vi "FPGA_1R_ADC_1W_DAC_2AI_Phaseunwrap_Oct.vi"() -> ()   [LabVIEW 2019]
uses:
  <vilib>/rvi/FXPMathLib/FxpSinAndCos/subVIs/nifxpmath_SinAndCos_SimConfig.ctl
  <vilib>/rvi/FXPMathLib/FxpAtan2/subVIs/nifxpmath_Atan2_SimConfig.ctl
  <vilib>/rvi/Emulation/niFpgaGetClockAttributes.vi
  <vilib>/rvi/Emulation/niFpgaSctlEmulationGetInTimedLoop.vi
  <vilib>/rvi/Emulation/niFpgaEmulationReportErrorSimple.vi
  <vilib>/rvi/eio/common/nirviEmuTemplateMethod_errors.vi
  <vilib>/rvi/Emulation/niFpgaCriticalErrorInLSC.vi
  <vilib>/rvi/FXPMathLib/FxpSinAndCos/simVIs/DllFxpSinAndCosTemp_sub.vi
  <vilib>/rvi/FXPMathLib/FxpAtan2/simVIs/DllFxpAtan2Temp_sub.vi
  <vilib>/eio/EIONode/EIONode.xnode
  <vilib>/rvi/FXPMathLib/basic elements/FxpAddSub/XNode/nifxpmath_AddSub.xnode
  <vilib>/rvi/FXPMathLib/FxpSinAndCos/XNode/nifxpmath_SinAndCos.xnode
  <vilib>/rvi/FXPMathLib/FxpMul/XNode/nifxpmath_Multiplier.xnode
  <vilib>/rvi/FXPMathLib/FxpSub/XNode/nifxpmath_Sub.xnode
  <vilib>/rvi/FXPMathLib/FxpAdd/XNode/nifxpmath_Add.xnode
  <vilib>/rvi/FXPMathLib/FxpAtan2/XNode/nifxpmath_Atan2.xnode
  <vilib>/rvi/FXPMathLib/basic elements/FxpDiscreteDelay/XNode/nifxpmath_DiscreteDelay.xnode
  <vilib>/rvi/FXPMathLib/sim/FxpSim.dll
panel:
  out "unwrapped phase":fxp<+/-,47,33>
  out "X":fxp<+/-,64,28>
  out "Y":fxp<+/-,64,28>
  in  "1/a":fxp<+/-,16,2>
  in  "1/b":fxp<+/-,16,2>
  in  "x0":fxp<+/-,16,2>
  in  "y0":fxp<+/-,16,2>
  in  "theta":fxp<+/-,16,2>
  out "IFO Loop ticks actual":u32
  in  "IFO Timer Ticks":u32 caption="IFO Loop ticks desired"
  out "n":i32
  out "PD2":u16
  in  "?":bool
  out "PD1":u16
  in  "DAQ stop":bool
  out "ADC Read":bool[](array[boolean])
  out "DAQ TICKS":u32
  in  "DAQ WAIT TICKS":u32=800
  in  "DAC 1 write":bool[](array[boolean])=[FALSE, FALSE, FALSE, FALSE, FALSE, FALSE, FALSE, FALSE, FALSE, FALSE, FALSE, FALSE, FALSE, FALSE, FALSE, FALSE]
  out "XFWD":bool
  out "XREV":bool
  out "YFWD":bool
  out "YREV":bool
  in  "Limit flag stop":bool
  in  "ENC stop":bool
  out "Encoder A Ref":bool
  out "Encoder B Ref":bool
  out "Encoder A":i32
  out "Encoder B":i32
  in  "2^n avg_window":i16=8
  out "ENCODER OVERFLOW":bool
  out "ENCODER TICKS":u32
  in  "ENCODER TICK SETPOINT":u32=8
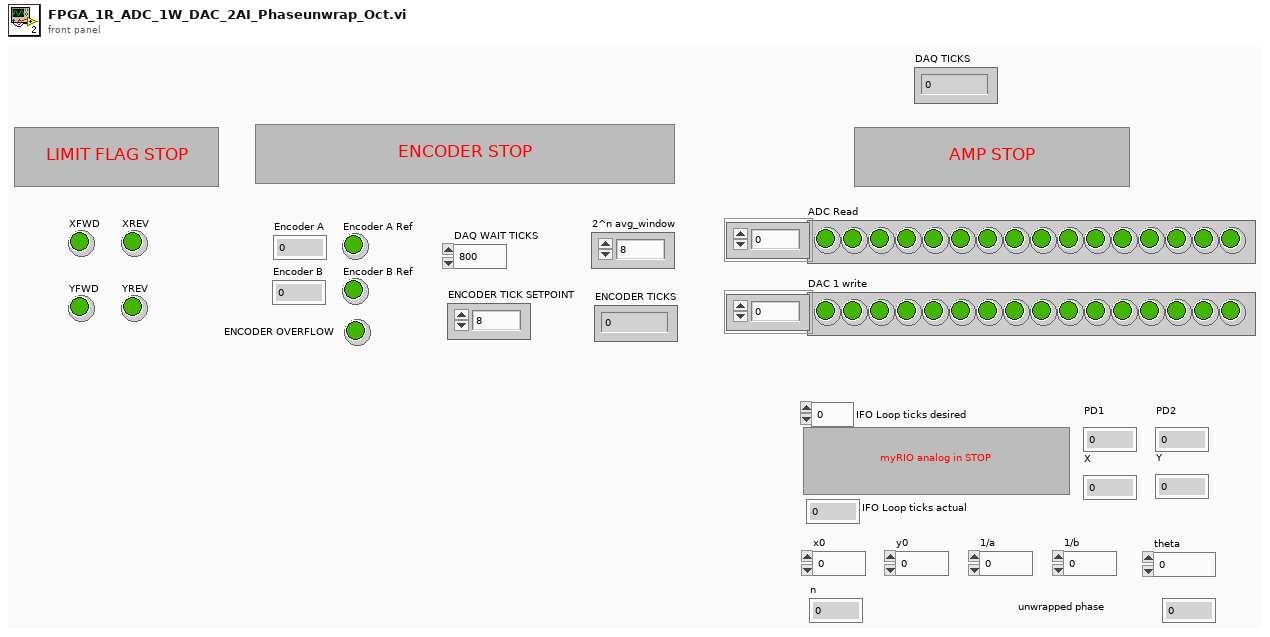
[diagram p1: front panel]
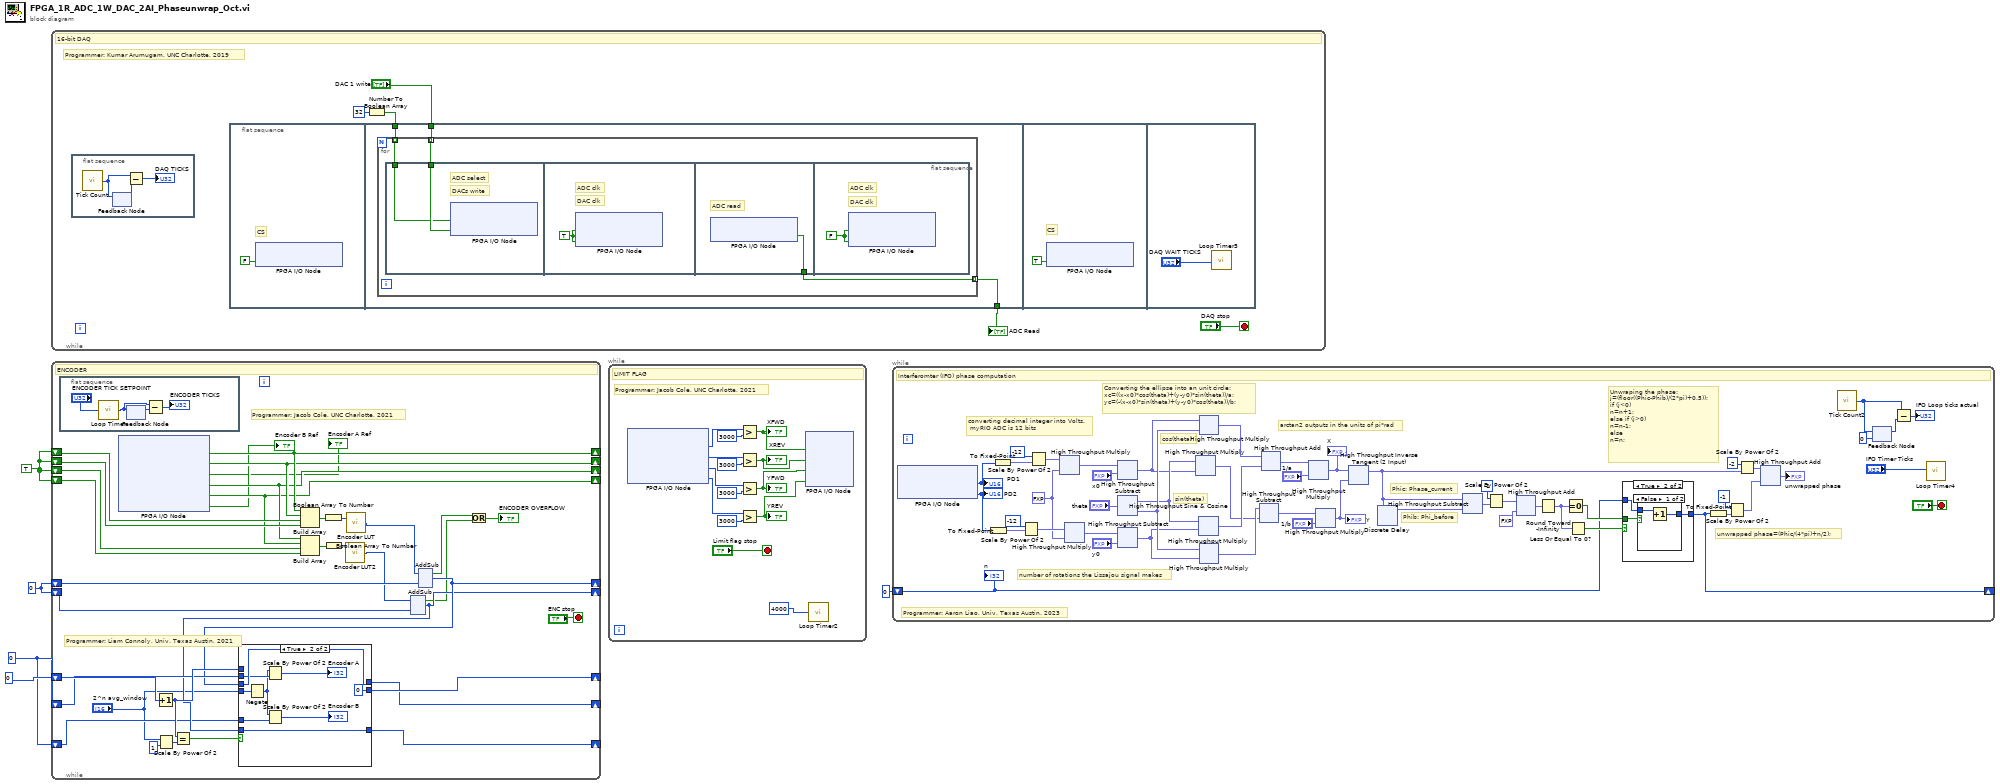
[diagram p0: block diagram]
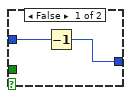
[diagram p2: hidden frame]
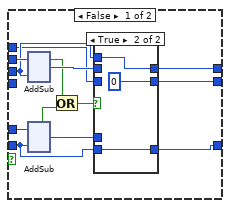
[diagram p4: hidden frame]
diagram:
  w2 = i64 0
  w4 = TRUE
  w5 = 0
  n1 = while {
    stop <- "DAQ stop" stop-if-true
    # "Programmer: Kumar Arumugam, UNC Charlotte, 2019"
    # "16-bit DAQ"
    n2 = flat-sequence {
      frame #0 {
        n3 = call "Tick Count"() -> ("Tick Count(Ticks)"=w27:u32)
        n4 = feedback #1() -> (w26:u32)  [unwired: 1 in]
        n5 = feedback-in #1(w27) -> ()
        n6 = Subtract(x=w27, y=w26) -> (x-y=→"DAQ TICKS":u32)
      }
    }
    n7 = flat-sequence {
      tunnel: "DAC 1 write" -> [w14]
      tunnel: w8 -> [w13]
      tunnel: [w12] -> w6
      frame #0 {
        # "CS"
        n8 = xnode "FPGA I/O Node"("ConnectorA/DIO4"=FALSE) -> ()  [unwired: 1 in, 1 out]
      }
      frame #1 {
        n9 = for {
          tunnel: w14 -> [w17] mode=indexing
          tunnel: [w16] -> w12 mode=indexing
          tunnel: w13 -> [w15] mode=indexing
          n10 = flat-sequence {
            tunnel: w17 -> [w19]
            tunnel: w15 -> [w18]
            tunnel: [w21] -> w16
            frame #0 {
              # "DACs write"
              # "ADC select"
              n11 = xnode "FPGA I/O Node"("ConnectorA/DIO2"=w18, "ConnectorA/DIO6"=w19) -> ()  [unwired: 2 in, 2 out]
            }
            frame #1 {
              w20 = TRUE ("ConnectorA/DIO3")
              # "DAC clk"
              # "ADC clk"
              n12 = xnode "FPGA I/O Node"("ConnectorA/DIO3"=w20, "ConnectorA/DIO5"=w20) -> ()  [unwired: 2 in, 2 out]
            }
            frame #2 {
              # "ADC read"
              n13 = xnode "FPGA I/O Node"() -> ("ConnectorA/DIO1"=w21:bool)  [unwired: 1 in, 1 out]
            }
            frame #3 {
              w22 = FALSE ("ConnectorA/DIO3")
              # "DAC clk"
              # "ADC clk"
              n14 = xnode "FPGA I/O Node"("ConnectorA/DIO3"=w22, "ConnectorA/DIO5"=w22) -> ()  [unwired: 2 in, 2 out]
            }
          }
        }
      }
      frame #2 {
        # "CS"
        n15 = xnode "FPGA I/O Node"("ConnectorA/DIO4"=TRUE) -> ()  [unwired: 1 in, 1 out]
      }
      frame #3 {
        n16 = call "Loop Timer3"("Count(Ticks)"="DAQ WAIT TICKS") -> ()  [unwired: 1 out]
      }
    }
    n17 = Number To Boolean Array(number=u16 32) -> (Boolean array=w8:bool[])
    "ADC Read" <- w6
  }
  n18 = while {
    shift-right: [w41] -> _
    shift-left: w5 -> [w39]
    shift-right: [w55] -> _
    shift-left: w4 -> [w61]
    shift-right: [w54] -> _
    shift-left: w4 -> [w58]
    shift-right: [w53] -> _
    shift-left: w4 -> [w57]
    shift-right: [w52] -> _
    shift-left: w4 -> [w56]
    shift-right: [w36] -> _
    shift-left: w5 -> [w37]
    shift-right: [w44] -> _
    shift-left: i16 0 -> [w47]
    shift-right: [w43] -> _
    shift-left: w2 -> [w42]
    shift-right: [w35] -> _
    shift-left: w2 -> [w34]
    stop <- "ENC stop" stop-if-true
    # "Programmer: Liam Connoly, Univ. Texas Austin, 2021"
    # "Programmer: Jacob Cole, UNC Charlotte, 2021"
    # "ENCODER"
    n19 = flat-sequence {
      frame #0 {
        n20 = call "Loop Timer"("Count(Ticks)"="ENCODER TICK SETPOINT") -> ("Tick Count(Ticks)"=w65:u32)
        n21 = feedback #2() -> (w64:u32)  [unwired: 1 in]
        n22 = feedback-in #2(w65) -> ()
        n23 = Subtract(x=w65, y=w64) -> (x-y=→"ENCODER TICKS":u32)
      }
    }
    n24 = xnode "FPGA I/O Node"() -> ("ConnectorA/DIO10"=w55:bool, "ConnectorA/DIO9"=w54:bool, "ConnectorA/DIO11"=→"Encoder A Ref":bool, "ConnectorA/DIO14"=w53:bool, "ConnectorA/DIO13"=w52:bool, "ConnectorA/DIO12"=→"Encoder B Ref":bool)  [unwired: 6 in, 6 out]
    n25 = Increment(x=w47) -> (x+1=w45:i16)
    n26 = Scale By Power Of 2(n="2^n avg_window", x=i64 1) -> (x*2^n=w31:i64)
    n27 = Equal?(x=w45, y=w31) -> (x = y?=w46:bool)
    n28 = Build Array(w55, w54, w61, w58) -> (w59:bool[])
    n29 = Build Array(w53, w52, w57, w56) -> (w60:bool[])
    n30 = Boolean Array To Number(Boolean array=w59) -> (number=w49:u8)
    n31 = Boolean Array To Number(Boolean array=w60) -> (number=w48:u8)
    n32 = call "Encoder LUT2"("address"=w48) -> ("data out"=w38:i32)  [unwired: 8 in]
    n33 = call "Encoder LUT"("address"=w49) -> ("data out"=w40:i32)  [unwired: 8 in]
    n34 = xnode "AddSub"("x"=w38, "y"=w37) -> ("s"=w36:i32, "overflow"=w29:bool)
    n35 = xnode "AddSub"("x"=w40, "y"=w39) -> ("s"=w41:i32, "overflow"=w30:bool)
    n36 = case shown="True" w46 {
      tunnel: w45 -> [w167 _]
      tunnel: [w168 i16 0] -> w44
      tunnel: w41 -> [w171 w289]
      tunnel: [w175 w289] -> w43
      tunnel: w42 -> [w177 w287]
      tunnel: w36 -> [w170 w288]
      tunnel: [w173 w288] -> w35
      tunnel: w34 -> [w176 w284]
      tunnel: "2^n avg_window" -> [_ w286]
      frame False {
        n37 = xnode "AddSub"("x"=w177, "y"=w171) -> ("s"=w174:i64, "overflow"=w166:bool)
        n38 = xnode "AddSub"("x"=w176, "y"=w170) -> ("s"=w172:i64, "overflow"=w165:bool)
        n39 = Or(x=w166, y=w165) -> (x .or. y?=w169:bool)
        n40 = case shown="True" w169 {
          tunnel: [w180 w183] -> w175
          tunnel: w174 -> [w180 _]
          tunnel: [w179 w182] -> w173
          tunnel: w172 -> [w179 _]
          tunnel: w171 -> [_ w183]
          tunnel: w170 -> [_ w182]
          tunnel: [w178 i16 0] -> w168
          tunnel: w167 -> [w178 _]
          frame False {
          }
          frame True {
          }
        }
      }
      frame True {
        n41 = Negate(x=w286) -> (-x=w283:i16)
        n42 = Scale By Power Of 2(n=w283, x=w287) -> (x*2^n=→"Encoder A":i64)
        n43 = Scale By Power Of 2(n=w283, x=w284) -> (x*2^n=→"Encoder B":i64)
      }
    }
    n44 = Or(x=w30, y=w29) -> (x .or. y?=→"ENCODER OVERFLOW":bool)
  }
  n45 = while {
    stop <- "Limit flag stop" stop-if-true
    # "Programmer: Jacob Cole, UNC Charlotte, 2021"
    # "LIMIT FLAG"
    n46 = xnode "FPGA I/O Node"() -> ("ConnectorA/AI0"=w300:u16, "ConnectorA/AI1"=w299:u16, "ConnectorA/AI2"=w298:u16, "ConnectorA/AI3"=w297:u16)  [unwired: 4 in, 4 out]
    n47 = Greater?(x=w300, y=u16 3000) -> (0:w294:bool)
    "XFWD" <- w294
    n48 = Greater?(x=w299, y=u16 3000) -> (0:w293:bool)
    "XREV" <- w293
    n49 = Greater?(x=w298, y=u16 3000) -> (0:w292:bool)
    "YFWD" <- w292
    n50 = Greater?(x=w297, y=u16 3000) -> (0:w291:bool)
    "YREV" <- w291
    n51 = xnode "FPGA I/O Node"("LED0"=w294, "LED1"=w293, "LED2"=w292, "LED3"=w291) -> ()  [unwired: 4 in, 4 out]
    n52 = call "Loop Timer2"("Count(Ticks)"=u32 4000) -> ()  [unwired: 1 out]
  }
  n53 = while {
    shift-right: [w333] -> _
    shift-left: 0 ("n") -> [w334]
    stop <- "?" stop-if-true
    w320 = fxp<+,16,5> 5.0 ("y")
    # "number of rotations the Lissajou signal makes"
    # "unwrapped phase=(Phic/(4*pi)+n/2);"
    # "Programmer: Aaron Liao, Univ. Texas Austin, 2023"
    # "Unwraping the phase:\nj=(floor((Phic-Phib)/(2*pi)+0.5));\nif (j<0)\nn=n+1;\nelse if (j>0)\nn=n-1;\nelse\nn=n;"
    # "arctan2 outputs in the units of pi*rad"
    # "Converting the ellipse into an unit circle:\nxc=((x-x0)*cos(theta)+(y-y0)*sin(theta))/a;\nyc=(-(x-x0)*sin(theta)+(y-y0)*cos(theta))/b;"
    # "converting decimal integer into Volts.\n myRIO ADC is 12 bits"
    # "Phic: Phase_current"
    # "Phib: Phi_before"
    # "cos(theta)"
    # "sin(theta)"
    # "Interferomter (IFO) phase computation"
    n54 = xnode "FPGA I/O Node"() -> ("ConnectorB/AI0"=w307:u16, "ConnectorB/AI1"=w308:u16)  [unwired: 2 in, 2 out]
    "PD1" <- w307
    "PD2" <- w308
    n55 = To Fixed-Point(number=w308) -> (fixed-point=w324:fxp<+,32,16>)  [unwired: 1 in]
    n56 = To Fixed-Point(number=w307) -> (fixed-point=w321:fxp<+,32,16>)  [unwired: 1 in]
    n57 = Scale By Power Of 2(n=i16 -12, x=w324) -> (x*2^n=w323:fxp<+,32,16>)
    n58 = Scale By Power Of 2(n=i16 -12, x=w321) -> (x*2^n=w319:fxp<+,32,16>)
    n59 = xnode ("High Throughput Multiply")("x"=w319, "y"=w320) -> ("x*y"=w318:fxp<+,48,21>)
    n60 = xnode ("High Throughput Multiply")("x"=w323, "y"=w320) -> ("x*y"=w353:fxp<+,48,21>)
    n61 = xnode "High Throughput Subtract"("x"=w318, "y"="x0") -> ("x-y"=w345:fxp<+/-,50,23>)
    n62 = xnode "High Throughput Sine & Cosine"("x (pi)"="theta") -> ("sin(x)"=w347:fxp<+/-,16,2>, "cos(x)"=w348:fxp<+/-,16,2>)
    n63 = xnode "High Throughput Subtract"("x"=w353, "y"="y0") -> ("x-y"=w346:fxp<+/-,50,23>)
    n64 = xnode ("High Throughput Multiply")("x"=w347, "y"=w345) -> ("x*y"=w343:fxp<+/-,64,25>)
    n65 = xnode ("High Throughput Multiply")("x"=w347, "y"=w346) -> ("x*y"=w351:fxp<+/-,64,25>)
    n66 = xnode ("High Throughput Multiply")("x"=w345, "y"=w348) -> ("x*y"=w354:fxp<+/-,64,25>)
    n67 = xnode ("High Throughput Multiply")("x"=w348, "y"=w346) -> ("x*y"=w344:fxp<+/-,64,25>)
    n68 = xnode "High Throughput Subtract"("x"=w344, "y"=w343) -> ("x-y"=w341:fxp<+/-,64,26>)
    n69 = xnode ("High Throughput Add")("x"=w354, "y"=w351) -> ("x+y"=w350:fxp<+/-,64,26>)
    n70 = xnode ("High Throughput Multiply")("x"=w350, "y"="1/a") -> ("x*y"=w317:fxp<+/-,64,28>)
    "X" <- w317
    n71 = xnode ("High Throughput Multiply")("x"=w341, "y"="1/b") -> ("x*y"=w316:fxp<+/-,64,28>)
    "Y" <- w316
    n72 = xnode "High Throughput Inverse Tangent (2 Input)"("y"=w317, "x"=w316) -> ("atan2(y,x) (pi)"=w312:fxp<+/-,16,2>)
    n73 = xnode ("Discrete Delay")("D"=w312) -> ("Q"=w340:fxp<+/-,16,2>)
    n74 = xnode "High Throughput Subtract"("x"=w312, "y"=w340) -> ("x-y"=w311:fxp<+/-,17,3>)
    n75 = Scale By Power Of 2(n=i16 -1, x=w311) -> (x*2^n=w310:fxp<+/-,17,3>)
    n76 = xnode ("High Throughput Add")("x"=w310, "y"=fxp<+/-,19,18> 0.5 ("x/y")) -> ("x+y"=w338:fxp<+/-,33,19>)
    n77 = Round Toward -Infinity(1:w338) -> (0:w336:fxp<+/-,19,19>)
    n78 = Equal To 0?(x=w336) -> (x = 0?=w335:bool)
    n79 = Less Or Equal To 0?(x=w336) -> (x <= 0?=w337:bool)
    n80 = case shown="True" w337 {
      tunnel: w335 -> [_ w361]
      tunnel: w334 -> [w358 w360]
      tunnel: [w357 w359] -> w333
      frame False {
        n81 = Decrement(x=w358) -> (x-1=w357:i32)
      }
      frame True {
        n82 = case shown="False" w361 {
          tunnel: w360 -> [w363 w364]
          tunnel: [w362 w364] -> w359
          frame False {
            n83 = Increment(x=w363) -> (x+1=w362:i32)
          }
          frame True {
          }
        }
      }
    }
    n84 = To Fixed-Point(number=w333) -> (fixed-point=w331:fxp<+/-,32,32>)  [unwired: 1 in]
    n85 = Scale By Power Of 2(n=i16 -1, x=w331) -> (x*2^n=w329:fxp<+/-,32,32>)
    n86 = Scale By Power Of 2(n=i16 -2, x=w312) -> (x*2^n=w314:fxp<+/-,16,2>)
    n87 = xnode ("High Throughput Add")("x"=w314, "y"=w329) -> ("x+y"=→"unwrapped phase":fxp<+/-,47,33>)
    n88 = call "Tick Count2"() -> ("Tick Count(Ticks)"=w328:u32)
    n89 = feedback #3(u32 0 ("Tick Count(Ticks)")) -> (w327:u32)
    n90 = feedback-in #3(w328) -> ()
    n91 = Subtract(x=w328, y=w327) -> (x-y=→"IFO Loop ticks actual":u32)
    n92 = call "Loop Timer4"("Count(Ticks)"="IFO Timer Ticks") -> ()  [unwired: 1 out]
    "n" <- w334
  }
